vi "Read ADC.vi"(8 "error in (no error)":errorcluster, 10 "ADC CH":dbl, 11 "Arduino in":refnum<class "Arduino.lvclass">) -> (0 "error out":errorcluster, 3 "Arduino out":refnum<class "Arduino.lvclass">)   [LabVIEW 2020, in "Arduino.lvclass"]
uses:
  Arduino.lvclass
  97330ff9-b66d-4380-9791-8744d3067609.vi
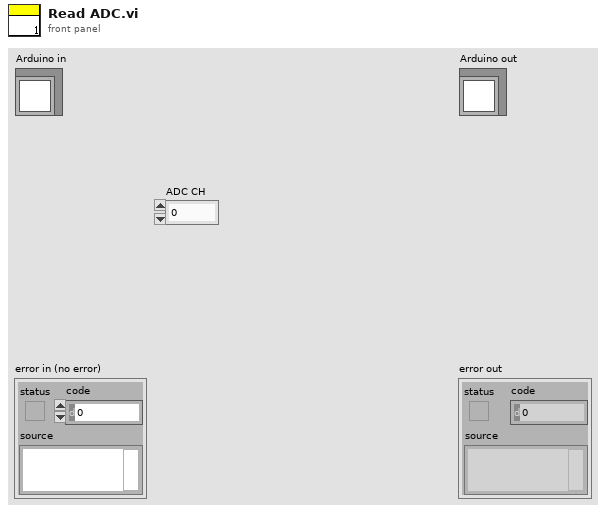
[diagram p1: front panel]
types:
  T1 = typedef "Serial Device.lvclass/serial device brand.ctl" = string
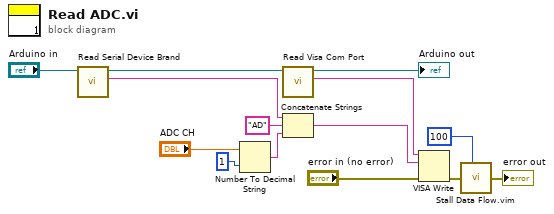
[diagram p0: block diagram]
diagram:
  n1 = call-dynamic "Read Serial Device Brand.vi"("Serial Device in"="Arduino in") -> ("Serial Device Brand"=w10:T1, "Serial Device out"=w11:refnum<class "Arduino.lvclass">)  [unwired: 8 in, 1 out]
  n2 = Number To Decimal String(number="ADC CH", width (-)=i16 1) -> (decimal integer string=w8:string)
  n3 = call-dynamic "Read Visa Com Port.vi"("Serial Device in"=w11) -> ("Visa Com Port"=w7:string, "Serial Device out"=→"Arduino out":refnum<class "Arduino.lvclass">)  [unwired: 8 in, 1 out]
  n4 = Concatenate Strings(w10, "AD" ("string"), w8) -> (w6:string)
  n5 = VISA Write(VISA resource name=w7, write buffer=w6, error in (no error)="error in (no error)") -> (error out=w3:errorcluster)  [unwired: 2 out]
  n6 = call "Stall Data Flow.vim"("value in"=w3, "milliseconds to wait"=u32 100) -> ("value out"=→"error out":errorcluster)  [unwired: 1 out]
